vi "get message components.vi"(11 "message":refnum<class "communicator message.lvclass">) -> (2 "data":variant, 3 "ID":string)   [LabVIEW 2015, in "communicator message.lvclass"]
uses:
  communicator message.lvclass
  communicator message.lvclass/communicator message.ctl
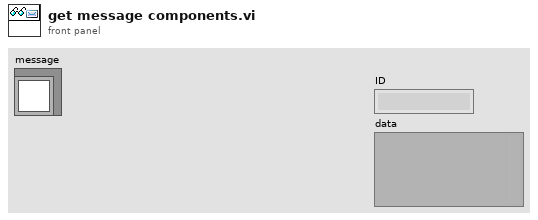
[diagram p1: front panel]
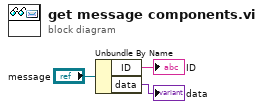
[diagram p0: block diagram]
diagram:
  n1 = Unbundle By Name("message") -> ("ID"=→"ID":string, "data"=→"data":variant)
